vi "SV Get Channels By Unit.vi"(4 "units to match":string[](array[string]), 5 "scaled signals [EU]":waveform(dbl)[](array[waveform])) -> (0 "matching channels [EU]":waveform(dbl)[](array[waveform]), 1 "number of matching channels":i32, 2 "scaled signals with matching channels deleted":waveform(dbl)[](array[waveform]))   [LabVIEW 2017]
uses:
  <vilib>/addons/_NISVFA/_Shared subVIs/Common/sv_Get NI Property Name String.vi
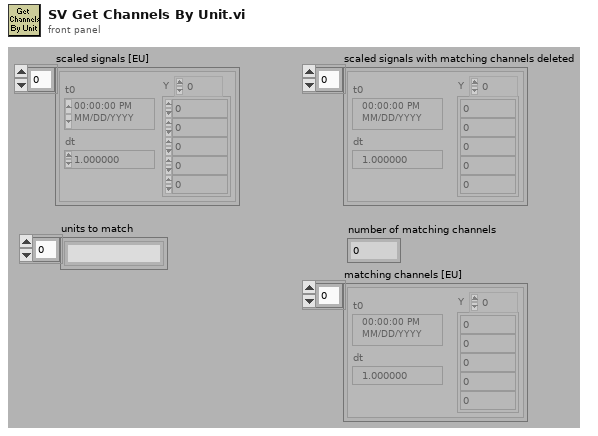
[diagram p1: front panel]
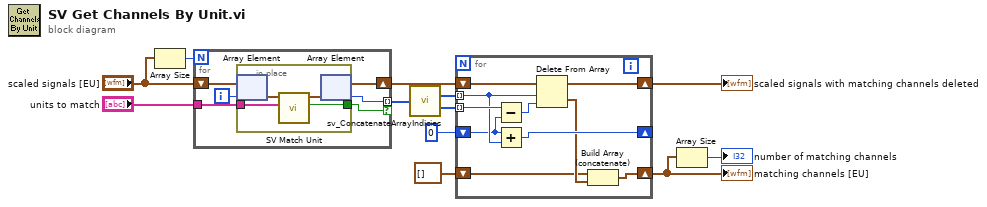
[diagram p0: block diagram]
diagram:
  n1 = Array Size(array="scaled signals [EU]") -> (size(s)=w3:i32)
  n2 = for {
    N: w3 -> [_]
    tunnel: "units to match" -> [w18]
    shift-right: [w16] -> w4
    shift-left: "scaled signals [EU]" -> [w17]
    tunnel: [w13] -> w1 mode=indexing if=w15
    i -> [w14]
    n3 = in-place {
      in-place-border: w18 -> [w22]
      in-place-border: [w19] -> w15
      n4 = in-place-array #1(w17, w14) -> (w21:waveform(dbl))
      n5 = call <vilib>:"SV Match Unit.vi"("Units to Match"=w22, "scaled signal [EU]"=w21) -> ("Found?"=w19:bool, "dup scaled signal [EU]"=w20:waveform(dbl))  [unwired: 6 in, 2 out]
      n6 = in-place-array #1(w20) -> (w16:waveform(dbl)[], w13:i32)
    }
  }
  n7 = call <vilib>:"sv_ConcatenateArrayIndicies.vi"("indices"=w1) -> ("subset lengths"=w8:i32[], "subset start indices"=w7:i32[])  [unwired: 13 in]
  n8 = for {
    shift-right: [w31] -> w9
    shift-left: w4 -> [w32]
    shift-right: [w23] -> w11
    shift-left: waveform(dbl)[] [] -> [w24]
    shift-right: [w29] -> _
    shift-left: 0 -> [w26]
    tunnel: w7 -> [w30] mode=indexing
    tunnel: w8 -> [w28] mode=indexing
    n9 = Subtract(x=w30, y=w26) -> (x-y=w27:i32)
    n10 = Add(x=w26, y=w28) -> (x+y=w29:i32)
    n11 = Delete From Array(array=w32, length=w28, index=w27) -> (deleted portion=w25:waveform(dbl)[], array with subset deleted=w31:waveform(dbl)[])
    n12 = Build Array (concatenate)(w24, w25) -> (w23:waveform(dbl)[])
  }
  "matching channels [EU]" <- w11
  "scaled signals with matching channels deleted" <- w9
  n13 = Array Size(array=w11) -> (size(s)=→"number of matching channels":i32)
